vi "Get Gyro Sensor.vi"() -> (2 "Robot Field Orientation (deg)":dbl)   [LabVIEW 2019]
uses:
  gyro sensor NavX/_TypeDefs/FRIC_navX_DeviceNumbersTypeDef.ctl
  <vilib>/Rock Robotics/Network Tables/NT Write Number.vi
  <vilib>/Rock Robotics/Network Tables/NT Read Number.vi
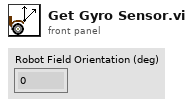
[diagram p1: front panel]
types:
  T1 = typedef "FRIC_navX_DeviceNumbersTypeDef.ctl" = enum16{"Dev0", "Dev1", "Dev2", "Dev3"}
  T2 = cluster{"Yaw":dbl, "Roll":dbl, "Pitch":dbl, "Heading":dbl, "Fused Heading":dbl}
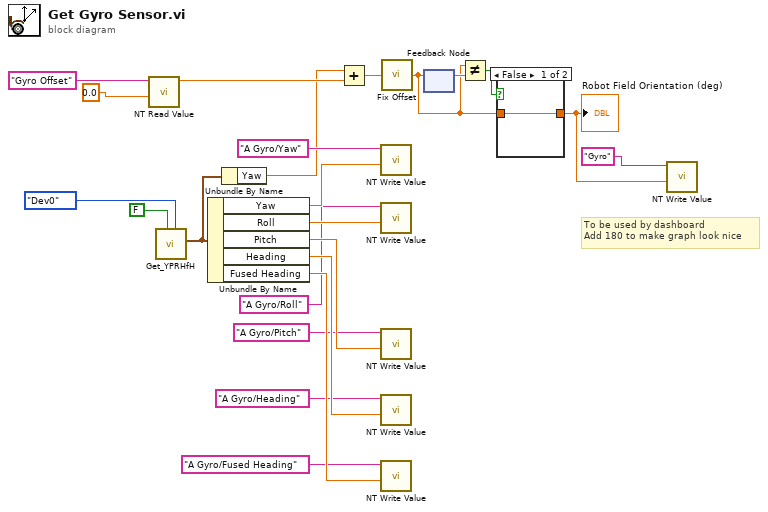
[diagram p0: block diagram]
diagram:
  # "To be used by dashboard\nAdd 180 to make graph look nice"
  n1 = call-poly <vilib>:"NT Read Value.vi"("Default Value"=0.0, "Name"="Gyro Offset") -> ("Numeric"=w8:dbl)  [unwired: 8 in, 1 out]
  n2 = call "Get_YPRHfH.vi"("Device Number"=FRIC_navX_DeviceNumbersTypeDef."Dev0", "Update"=FALSE) -> ("YRPHfH"=w9:T2)  [unwired: 9 in]
  n3 = Unbundle By Name(w9) -> ("Yaw"=w22:dbl, "Roll"=w21:dbl, "Pitch"=w20:dbl, "Heading"=w19:dbl, "Fused Heading"=w18:dbl)
  n4 = Unbundle By Name(w9) -> ("Yaw"=w5:dbl)
  n5 = Add(x=w5, y=w8) -> (x+y=w10:dbl)
  n6 = call-poly <vilib>:"NT Write Value.vi"("Numeric"=w22, "Name"="A Gyro/Yaw") -> ()  [unwired: 9 in, 1 out]
  n7 = call-poly <vilib>:"NT Write Value.vi"("Numeric"=w21, "Name"="A Gyro/Roll") -> ()  [unwired: 9 in, 1 out]
  n8 = call-poly <vilib>:"NT Write Value.vi"("Numeric"=w20, "Name"="A Gyro/Pitch") -> ()  [unwired: 9 in, 1 out]
  n9 = call-poly <vilib>:"NT Write Value.vi"("Numeric"=w19, "Name"="A Gyro/Heading") -> ()  [unwired: 9 in, 1 out]
  n10 = call-poly <vilib>:"NT Write Value.vi"("Numeric"=w18, "Name"="A Gyro/Fused Heading") -> ()  [unwired: 9 in, 1 out]
  n11 = call "Fix Offset.vi"("Input Angle"=w10) -> ("Output Angle"=w2:dbl)
  n12 = feedback #1() -> (w4:dbl)  [unwired: 1 in]
  n13 = feedback-in #1(w2) -> ()
  n14 = Not Equal?(x=w2, y=w4) -> (x != y?=w3:bool)
  n15 = case shown="False" w3 {
    tunnel: w2 -> [w24 w25]
    tunnel: [w24 w25] -> w1
    frame False {
    }
    frame True {
    }
  }
  "Robot Field Orientation (deg)" <- w1
  n16 = call-poly <vilib>:"NT Write Value.vi"("Numeric"=w1, "Name"="Gyro") -> ()  [unwired: 9 in, 1 out]
